vi "Dashboard Main.vi"() -> ()   [LabVIEW 2015]
uses:
  <vilib>/event_ctls.llb/eventvkey.ctl
  <vilib>/Utility/config.llb/NI_LVConfig.lvlib
  <vilib>/Utility/config.llb/Write Key (I32).vi
  <vilib>/Rock Robotics/WPI/Dashboard/WPI_DashboardLogging Global.vi
  <vilib>/Utility/config.llb/Write Key (String).vi
  <vilib>/Rock Robotics/Network Tables/NT Read Numeric Array.vi
  <vilib>/Utility/miscctls.llb/LVRowAndColumnTypeDef.ctl
  <vilib>/Rock Robotics/Network Tables/NT Write Boolean.vi
  <vilib>/Rock Robotics/Network Tables/NT Read Boolean.vi
panel:
  in  "TCP":refnum<k5>
  in  "Rec Mode":enum32{"Stop", "Record", "Playback"}(radio)
  in  "Vision":u16(ring) items=["Camera Off", "USB Camera SW", "USB Camera HW", "IP Camera"]
  out "Camera IP":string
  out "Image Message":string="Timeout in Camera Communications"
  in  "Dashboard Tab":T1(tab)
  in  "Select Auto":string(combo)
  out "NT Connection":bool
  in  "Camera Settings":T2={"Frame Rate"=30, "Compression"=30, "Size"=1} {"Frame Rate" scale=1.0..30.0; "Size" items=["640x480", "320x240", "160x120"]}
  out "MotorChart R":cluster{"Numeric":dbl, "Numeric":dbl}(graph)
  out "MotorChart L":T3(graph)
  out "MotorSliders R":cluster{"MotorSlide1":dbl, "MotorSlide2":dbl} {"MotorSlide2" scale=-1.0..1.0 scale format="%#_2e"; "MotorSlide1" scale=-1.0..1.0 scale format="%#_2e"}
  out "MotorSliders L":T4 {"MotorSlide4 2" scale=0.0..14.0 scale format="%#_2e"; "MotorSlide2" scale=-1.0..1.0 scale format="%#_2e"; "MotorSlide1" scale=-1.0..1.0 scale format="%#_2e"}
  out "Gyro":dbl(knob) scale=0.0..360.0
  out "JS1 Z":dbl(slide) scale=-1.0..1.0 scale format="%#_2e"
  out "JS1 Graph":cluster{"X":dbl, "Y":dbl}[](graph)
  out "JS1 Buttons":T5
  out "JS2 Z":dbl(slide) scale=-1.0..1.0 scale format="%#_2e"
  out "JS2 Graph":cluster{"X":dbl, "Y":dbl}[](graph)
  out "JS2 Buttons":T5
  out "Mode":T6(ring)=enum."Auto Disabled"
  in  "DB Camera Config":bool
  out "fps":dbl format="%#.1g"
  out "Mbps":dbl format="%#.1g"
  out "Mbps LED":bool
  in  "DB/String 9":string
  in  "DB/String 8":string
  in  "DB/String 7":string
  in  "DB/String 6":string
  in  "DB/String 5":string
  in  "DB/String 4":string
  in  "DB/String 3":string
  in  "DB/String 2":string
  in  "DB/String 1":string
  in  "DB/String 0":string
  in  "DB/Slider 0":dbl(slide) scale=0.0..5.0
  in  "DB/Slider 1":dbl(slide) scale=0.0..5.0
  in  "DB/Slider 2":dbl(slide) scale=0.0..5.0
  in  "DB/Slider 3":dbl(slide) scale=0.0..5.0
  out "DB/LED 3":bool
  out "DB/LED 2":bool
  out "DB/LED 1":bool
  out "DB/LED 0":bool
  in  "DB/Button 3":bool
  in  "DB/Button 2":bool
  in  "DB/Button 1":bool
  in  "DB/Button 0":bool caption="New Name"
  out "Meow2":bool
  in  "Meow":bool
  in  "Test Slider":dbl(slide) scale=0.0..100.0 scale format="%#_3g"
  in  "On/Off":bool caption="Solenoid"
  in  "Test Name":u16(ring) items=["Select the test to run..."]
  in  "Test Tree":string(tree)
  in  "Motor":cluster{"Value":dbl, "Enable":bool} {"Value" scale=-1.0..1.0 scale format="%#_3g"}
  out "Progress":T7 {"Test Progress" scale=0.0..100.0}
  in  "Rev/Fwd":cluster{"Forward":bool, "Reverse":bool}
  in  "Test Ring":u16(ring) items=["Monochrome", "Color"]
  out "Cmd Status":string
  in  "Execute Command":bool
  in  "Command Params":string[][](table)
  in  "Command Selection":i32(listbox)
  in  "CheckList":i32(listbox)
  out "Tree":string(tree)
  out "Camera Image":T8(plugin-control)
  out "Background":bool
  # "Left"
  # "Front"
  # "Right"
  # "Battery"
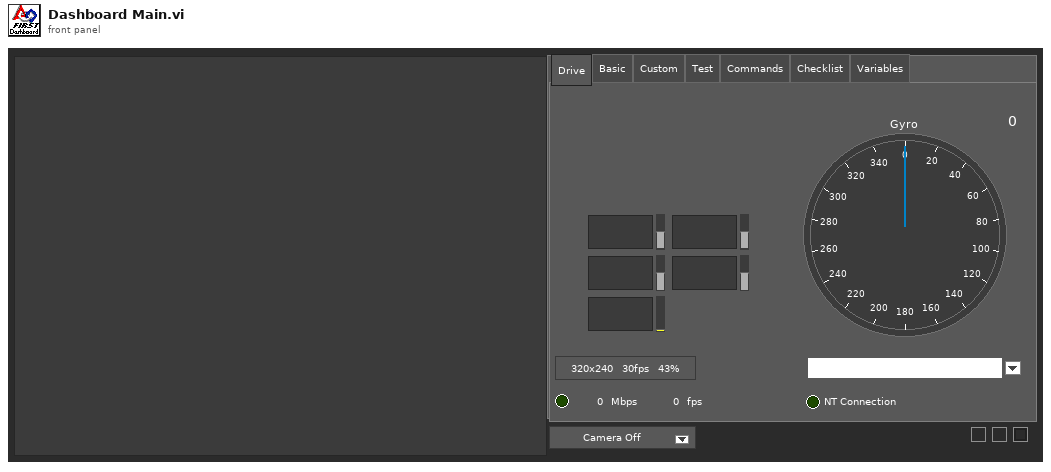
[diagram p1: front panel]
types:
  T1 = enum32{"Drive", "Basic", "Custom", "Test", "Commands", "Checklist", "Variables"}
  T2 = cluster{"Frame Rate":i32, "Compression":i32, "Size":u16}
  T3 = cluster{"Numeric":dbl, "Numeric":dbl, "Battery V":dbl}
  T4 = cluster{"MotorSlide1":dbl, "MotorSlide2":dbl, "MotorSlide4 2":dbl}
  T5 = cluster{bool, bool, bool, bool, bool, bool, bool, bool, bool, bool, bool, bool}
  T6 = enum8{"Tele-Op Disabled", "Tele-Op Enabled", "Auto Disabled", "Auto Enabled", "Test Disabled", "Test Enabled", "Disconnected", "No Code", "E-Stop"}
  T7 = cluster{"Test Progress":u8, "Test Progress Text":string}
  T8 = typedef "IMAQ Image.ctl" = refnum<image>
  T9 = cluster{"IDs":cluster{"RPC field ID":u16, "Unique ID":u16}, "String":string}
  T10 = enum32{"Drive", "Basic", "Custom", "Test", "Checklist", "Variables"}
  T11 = typedef "Image Type" = u32
  T12 = cluster{"Camera Image":refnum<vi>, "Dashboard Tab":refnum<vi>, "Background":refnum<vi>, "Vision":refnum<vi>, "Rec Mode":refnum<vi>, "Test Slider":refnum<vi>, "On/Off ":refnum<vi>, "Test Ring":refnum<vi>, "Rev/Fwd":refnum<vi>, "Test Name":refnum<vi>, "Motor":refnum<vi>, "Progress":refnum<vi>, "CheckList":refnum<vi>, "Tree":refnum<vi>, "Test Tree":refnum<vi>, "Command Params":refnum<vi>, "Command Selection":refnum<vi>, "Execute Command":refnum<vi>, "Cmd Status":refnum<vi>}
  T13 = cluster{"Error Strings":string, "Disable Counts":cluster{u16, u16}, "Rail Faults":cluster{u16, u16, u16}, "Robot IP":string, "DB Mode":u8, "Event Info":cluster{"Name":string, "Type":u8, "Number":u16, "Replay":u8}, "Camera Addr":string}
  T14 = cluster{"Storage":cluster{"Disk Free":u64, "RAM Block":u32, "RAM free":u32}, "CPU Utilization":cluster{"CPU % ISR":sgl, "CPU % Time Crit":sgl, "CPU % Timed Str":sgl, "CPU % High":sgl, "CPU % Above":sgl, "CPU % Normal":sgl, "CPU % Low":sgl}, "CAN":cluster{"% Bus Utilization":sgl, "Bus Off Cnt":u32, "TX_FIFO Full Cnt":u32, "Receive Error Cnt":u8, "Transmit Error Cnt":u8}, "HID":cluster{"HID Outputs":u32, "Rumble Low":u16, "Rumble High":u16}[]}
  T15 = cluster{"Status bits":cluster{"Test Mode":bool, "Autonomous":bool, "Enabled":bool, "Code Start":bool, "Brownout":bool, "Reserved 2":bool, "Reserved 3":bool, "E-Stop":bool}, "Code Trace":cluster{"Disabled":bool, "TeleOp":bool, "Auto":bool, "Test":bool}, "Controller Type":enum16{"unknown", "cRIO", "roboRio"}, "Code?":enum16{"unknown", "noCode", "code"}, "Battery V":dbl}
  T16 = cluster{"Control Bits":cluster{"TestMode":bool, "Autonomous":bool, "Enabled":bool, "FMS Present":bool, bool, bool, bool, "E-Stop":bool}, "Team Station ":u8, "Countdown":sgl, "Joystick Values":cluster{"Axes":dbl[], "Buttons":bool[], "POVs":i16[]}[]}
  T17 = cluster{"Axes":dbl[], "Buttons":bool[], "POVs":i16[]}[]
  T18 = cluster{"Axes":dbl[], "Buttons":bool[], "POVs":i16[]}
  T19 = cluster{"Buttons[0]":bool, "Buttons[1]":bool, "Buttons[2]":bool, "Buttons[3]":bool, "Buttons[4]":bool, "Buttons[5]":bool, "Buttons[6]":bool, "Buttons[7]":bool, "Buttons[8]":bool, "Buttons[9]":bool, "Buttons[10]":bool, "Buttons[11]":bool}
  T20 = typedef "NI_LVConfig.lvlib/Config Data RefNum.ctl" = refnum<k1>
  T21 = cluster{"Operation":enum16{"Update", "Clear"}, "Color Box":u32}[]
  T22 = typedef "eventvkey.ctl" = enum16{"ASCII", "Enter", "Return", "Shift", "Ctrl", "Alt", "Cmd", "Opt", "Caps", "NumLock", "Clear", "Break", "Up", "Down", "Left", "Right", "Insert", "Delete", "Home", "End", "PageUp", "PageDown", "Escape", "Help", "Pause", "ScrollLock", "F1", "F2", "F3", "F4", "F5", "F6", "F7", "F8", "F9", "F10", "F11", "F12", "F13", "F14", "F15", "F16", "F17", "F18", "F19", "F20", "F21", "F22", "F23", "F24", "Play", "VolumeUp", "VolumeDown", "Mute", "Two Byte Char"}
  T23 = cluster{"Image Size":bool, "Image Type":bool, "Pixel Value":bool, "ROI Information":bool, "Zoom Factor":bool}
  T24 = enum8{"Enabled", "Disabled", "Disabled and Grayed Out"}
  T25 = cluster{"Operation":enum16{"Update", "Clear"}, "Color Box":u32}
  T26 = typedef "LVRowAndColumnTypeDef.ctl" = cluster{"Row":i32, "Column":i32}
  T27 = cluster{"Shift":bool, "Ctrl":bool, "Alt":bool, "Cmd":bool, "Opt":bool}
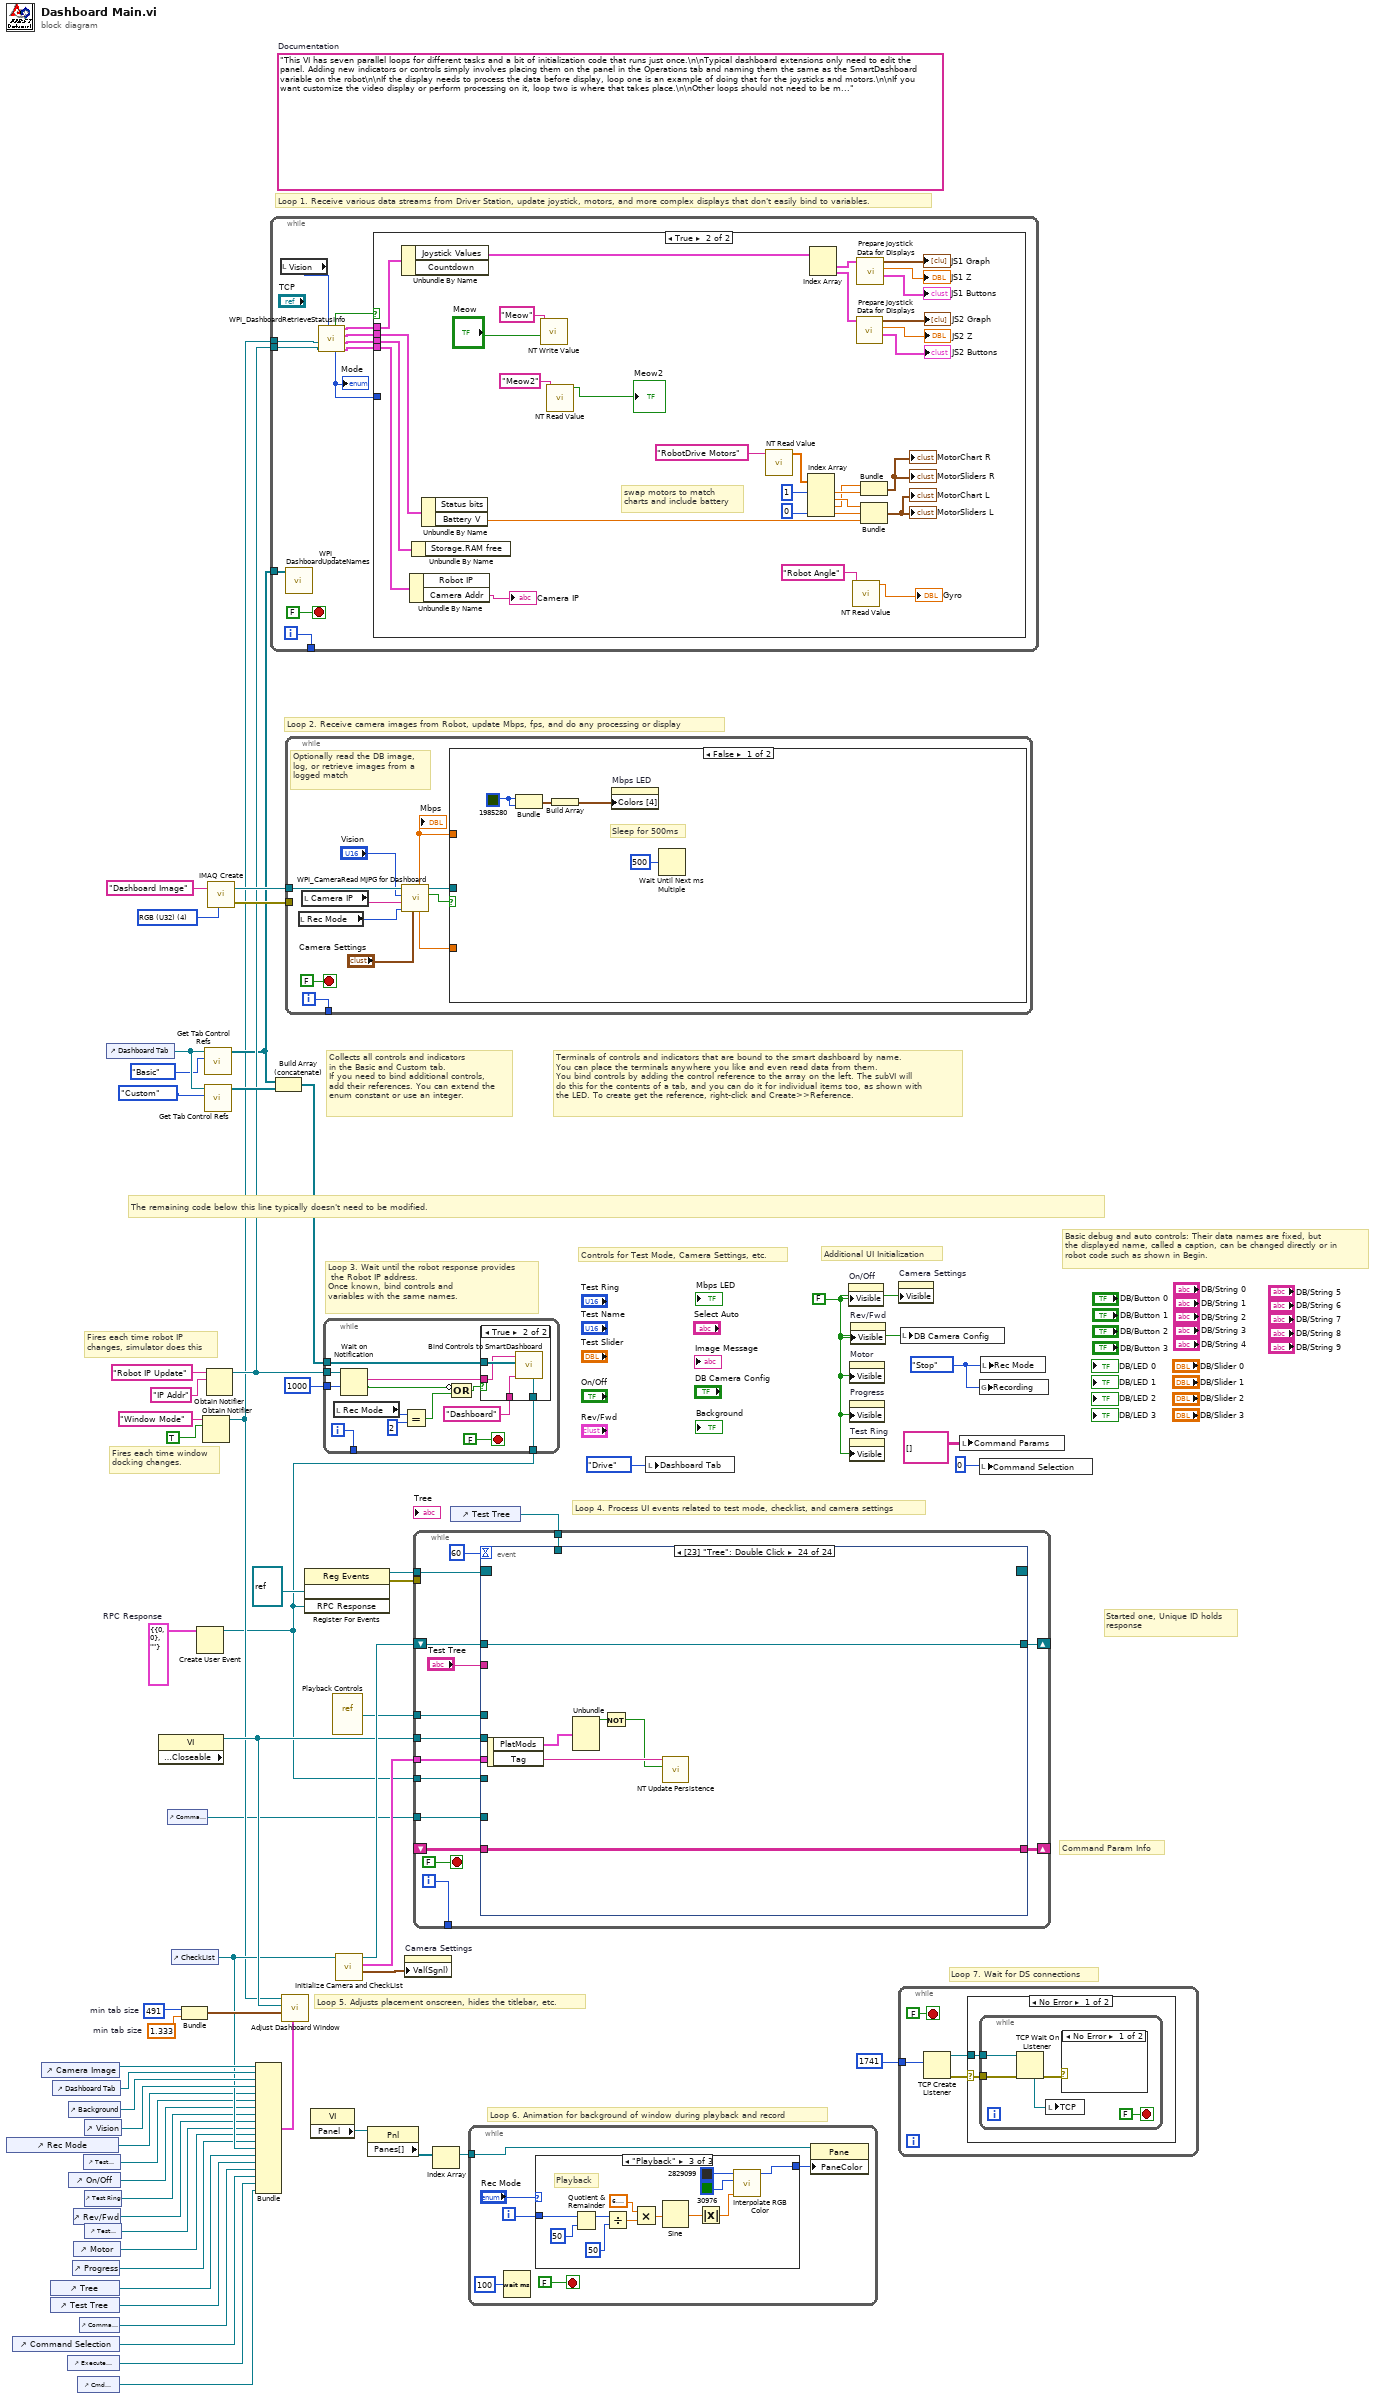
[diagram p0: block diagram]
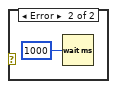
[diagram p2: hidden frame]
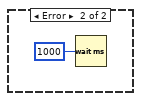
[diagram p3: hidden frame]
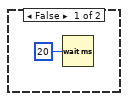
[diagram p4: hidden frame]
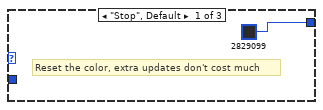
[diagram p5: hidden frame]
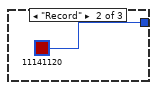
[diagram p6: hidden frame]
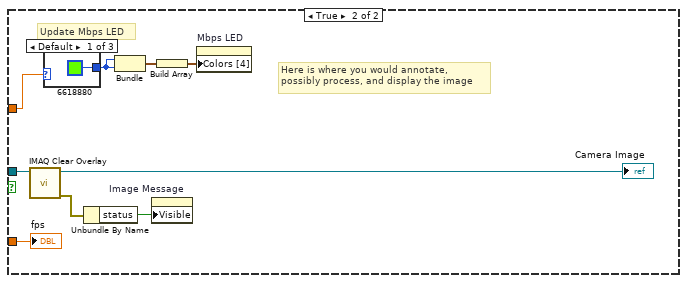
[diagram p8: hidden frame]
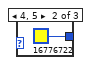
[diagram p9: hidden frame]
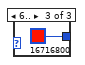
[diagram p10: hidden frame]
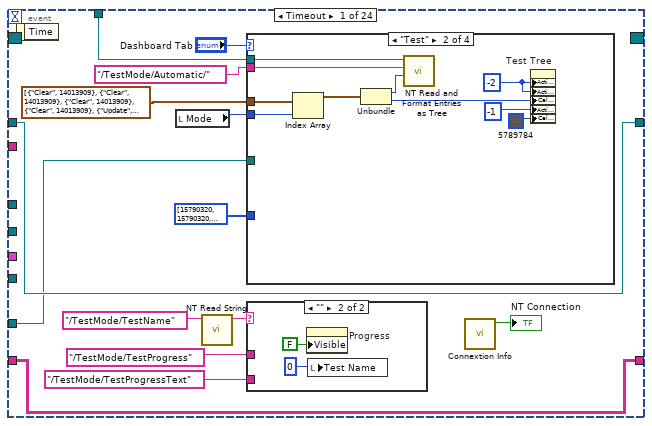
[diagram p11: hidden frame]
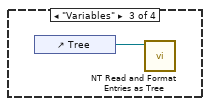
[diagram p13: hidden frame]
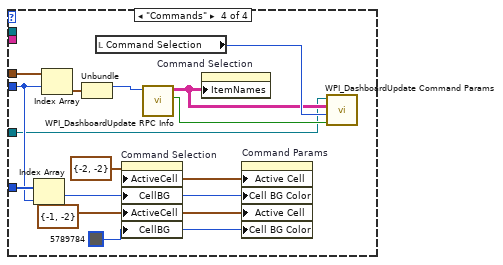
[diagram p14: hidden frame]
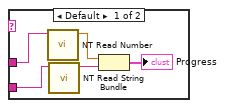
[diagram p15: hidden frame]
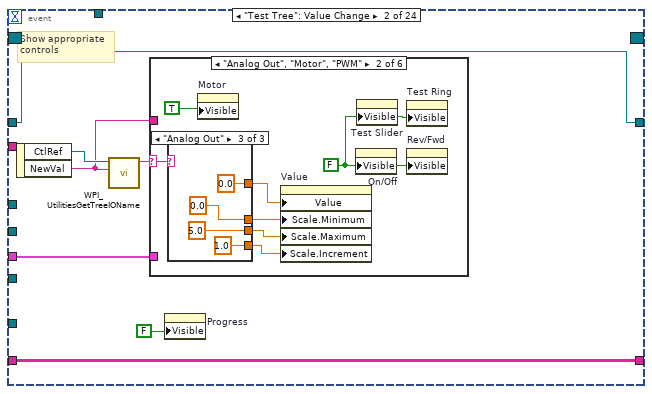
[diagram p16: hidden frame]
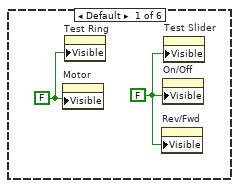
[diagram p17: hidden frame]
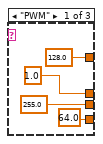
[diagram p18: hidden frame]
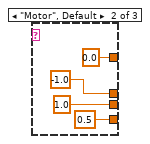
[diagram p19: hidden frame]
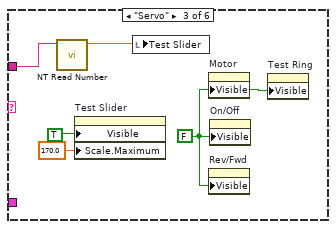
[diagram p20: hidden frame]
diagram:
  w7 = T9 {"IDs"={"RPC field ID"=0, "Unique ID"=0}, "String"=""}  # RPC Response
  w33 = 491  # min tab size
  w32 = 1.333  # min tab size
  w41 = enum32{"Stop", "Record", "Playback"}."Stop" ("Rec Mode")
  w15 = FALSE ("Visible")
  (unwired) "This VI has seven parallel loops for different tasks and a bit of initialization code that runs just once.\n\nTypical dashboard extensions only need to edit the panel. Adding new indicators or controls simply involves placing them on the panel in the Operations tab and naming them the same as the SmartDashboard variable on the robot\n\nIf the display needs to process the data before display, loop one is an example of doing that for the joysticks and motors.\n\nIf you want customize the video display or perform processing on it, loop two is where that takes place.\n\nOther loops should not need to be modified. They are pretty standard, and document the task they perform."  # Documentation
  w61 = T11 4 items=["Grayscale (U8)", "Grayscale (I16)", "Grayscale (SGL)", "Complex (CSG)", "RGB (U32)", "HSL (U32)", "RGB (U64)"] ("Image Type")
  # "Command Param Info"
  # "Started one, Unique ID holds\nresponse"
  # "Loop 7. Wait for DS connections"
  # "Basic debug and auto controls: Their data names are fixed, but\nthe displayed name, called a caption, can be changed directly or in\nrobot code such as shown in Begin."
  # "Controls for Test Mode, Camera Settings, etc."
  # "Additional UI Initialization"
  # "Loop 6. Animation for background of window during playback and record"
  # "Fires each time robot IP\nchanges, simulator does this"
  # "Fires each time window\ndocking changes."
  # "Collects all controls and indicators\nin the Basic and Custom tab.\nIf you need to bind additional controls,\nadd their references. You can extend the\nenum constant or use an integer."
  # "The remaining code below this line typically doesn't need to be modified."
  # "Loop 4. Process UI events related to test mode, checklist, and camera settings"
  # "Terminals of controls and indicators that are bound to the smart dashboard by name.\nYou can place the terminals anywhere you like and even read data from them.\nYou bind controls by adding the control reference to the array on the left. The subVI will\ndo this for the contents of a tab, and you can do it for individual items too, as shown with\nthe LED. To create get the reference, right-click and Create>>Reference."
  # "Loop 3. Wait until the robot response provides\n the Robot IP address.\nOnce known, bind controls and\nvariables with the same names."
  # "Loop 5. Adjusts placement onscreen, hides the titlebar, etc."
  # "Loop 1. Receive various data streams from Driver Station, update joystick, motors, and more complex displays that don't easily bind to variables."
  # "Loop 2. Receive camera images from Robot, update Mbps, fps, and do any processing or display"
  n1 = control-ref of="Rec Mode"() -> (w21:refnum<vi>)
  n2 = control-ref of="Command Selection"() -> (w6:refnum<vi>)
  n3 = control-ref of="Camera Image"() -> (w36:refnum<vi>)
  n4 = control-ref of="Tree"() -> (w25:refnum<vi>)
  n5 = control-ref of="Test Tree"() -> (w24:refnum<vi>)
  n6 = control-ref of="Dashboard Tab"() -> (w35:refnum<vi>)
  n7 = control-ref of="Execute Command"() -> (w8:refnum<vi>)
  n8 = control-ref of="Background"() -> (w30:refnum<vi>)
  n9 = control-ref of="On/Off"() -> (w19:refnum<vi>)
  n10 = control-ref of="Progress"() -> (w16:refnum<vi>)
  n11 = control-ref of="Rev/Fwd"() -> (w17:refnum<vi>)
  n12 = control-ref of="Motor"() -> (w22:refnum<vi>)
  n13 = control-ref of="Cmd Status"() -> (w2:refnum<vi>)
  n14 = control-ref of="Command Params"() -> (w9:refnum<vi>)
  n15 = control-ref of="Test Slider"() -> (w20:refnum<vi>)
  n16 = control-ref of="Vision"() -> (w34:refnum<vi>)
  n17 = control-ref of="Test Ring"() -> (w18:refnum<vi>)
  n18 = control-ref of="Test Name"() -> (w23:refnum<vi>)
  n19 = control-ref of="Dashboard Tab"() -> (w39:refnum<vi>)
  n20 = property class="VI" props=["Front Panel.Closeable"]() -> (reference out=w40:refnum<vi>)  [unwired: 2 in, 2 out]
  n21 = control-ref of="Command Params"() -> (w1:refnum<vi>)
  n22 = control-ref of="CheckList"() -> (w26:refnum<vi>)
  n23 = Bundle("min tab size"=w33, "min tab size"=w32) -> (w31:cluster{"min tab size":i32, "min tab size":dbl})  [unwired: 1 in]
  n24 = Create User Event(user event datatype=w7) -> (user event=w3:refnum<user-event>)  [unwired: 1 in, 1 out]
  n25 = Obtain Notifier(name (unnamed)="Window Mode", notification data type=TRUE) -> (notifier out=w12:refnum<notifier>)  [unwired: 2 in, 2 out]
  n26 = call <vilib>:"Get Tab Control Refs.vi"("Page Index"=T10."Basic" ("Dashboard Tab"), "TabControl in"=w39) -> ("ControlsOnPage"=w13:refnum<vi>[])  [unwired: 9 in]
  n27 = call <vilib>:"Get Tab Control Refs.vi"("Page Index"=T10."Custom" ("Dashboard Tab"), "TabControl in"=w39) -> ("ControlsOnPage"=w38:refnum<vi>[])  [unwired: 9 in]
  n28 = Obtain Notifier(name (unnamed)="Robot IP Update", notification data type="IP Addr" ("name (unnamed)")) -> (notifier out=w14:refnum<notifier>)  [unwired: 2 in, 2 out]
  n29 = call "IMAQ Create"("Image Name"="Dashboard Image", "Image Type"=w61) -> ("New Image"=w59:T8, "error out"=w58:errorcluster)  [unwired: 2 in, 1 out]
  n30 = Bundle("Camera Image"=w36, "Dashboard Tab"=w35, "Background"=w30, "Vision"=w34, "Rec Mode"=w21, "Test Slider"=w20, "On/Off"=w19, "Test Ring"=w18, "Rev/Fwd"=w17, "Test Name"=w23, "Motor"=w22, "Progress"=w16, "CheckList"=w26, "Tree"=w25, "Test Tree"=w24, "Command Params"=w9, "Command Selection"=w6, "Execute Command"=w8, "Cmd Status"=w2) -> (w27:T12)  [unwired: 1 in]
  n31 = while {
    tunnel: [w72] -> _
    tunnel: w14 -> [w63]
    tunnel: w13 -> [w71]
    tunnel: w12 -> [w62]
    i -> [w72]
    stop <- FALSE stop-if-true
    n32 = local read "Vision"() -> (w70:u16)
    n33 = call <vilib>:"WPI_DashboardUpdateNames.vi"("Controls on Tab"=w71) -> ()  [unwired: 11 in]
    n34 = call <vilib>:"WPI_DashboardRetrieveStatusInfo.vi"("Vision"=w70, "Binding Refnum"=w63, "Window Mode Notifier"=w62) -> ("Power and Errors"=w65:T13, "Robot Metrics"=w66:T14, "Status Info"=w67:T15, "Control Info"=w68:T16, "Robot Mode"=w64:T6, "Process?"=w69:bool)  [unwired: 3 in]
    "Mode" <- w64
    n35 = case shown="True" w69 {
      tunnel: w67 -> [_ w105]
      tunnel: w66 -> [_ w104]
      tunnel: w68 -> [_ w103]
      tunnel: w65 -> [_ w102]
      tunnel: w64 -> [_ _]
      frame False {
        n36 = Wait (ms)(milliseconds to wait=u32 20) -> ()  [unwired: 1 out]
      }
      frame True {
        # "swap motors to match\ncharts and include battery"
        n37 = Unbundle By Name(w103) -> ("Joystick Values"=w92:T17)  [unwired: 1 out]
        n38 = Unbundle By Name(w102) -> ("Camera Addr"=→"Camera IP":string)  [unwired: 1 out]
        n39 = Unbundle By Name(w104) -> ()  [unwired: 1 out]
        n40 = Unbundle By Name(w105) -> ("Battery V"=w93:dbl)  [unwired: 1 out]
        n41 = call-poly <vilib>:"NT Write Value.vi"("Boolean"="Meow", "Name"="Meow") -> ()  [unwired: 9 in, 1 out]
        n42 = call-poly <vilib>:"NT Read Value.vi"("Name"="Meow2") -> ("Boolean"=→"Meow2":bool)  [unwired: 9 in, 1 out]
        n43 = call-poly <vilib>:"NT Read Value.vi"("Name"="RobotDrive Motors") -> ("Numeric Array"=w81:dbl[])  [unwired: 9 in, 1 out]
        n44 = Index Array(array=w81, index #1=1, index #4=0) -> (element #1=w97:dbl, element #2=w98:dbl, element #3=w96:dbl, element #4=w101:dbl)  [unwired: 2 in]
        n45 = Index Array(array=w92) -> (element #1=w91:T18, element #2=w86:T18)  [unwired: 2 in]
        n46 = call-poly <vilib>:"NT Read Value.vi"("Name"="Robot Angle") -> ("Numeric"=→"Gyro":dbl)  [unwired: 9 in, 1 out]
        n47 = call "Prepare Joystick Data for Displays.vi"("Joystick Values"=w86) -> ("Buttons"=→"JS2 Buttons":T19, "Z Axis"=→"JS2 Z":dbl, "Cartesian Data"=→"JS2 Graph":cluster{"X axis":dbl, "X axis":dbl}[])  [unwired: 8 in]
        n48 = call "Prepare Joystick Data for Displays.vi"("Joystick Values"=w91) -> ("Buttons"=→"JS1 Buttons":T19, "Z Axis"=→"JS1 Z":dbl, "Cartesian Data"=→"JS1 Graph":cluster{"X axis":dbl, "X axis":dbl}[])  [unwired: 8 in]
        n49 = Bundle("Numeric"=w96, "Numeric"=w97) -> (→"MotorChart R" →"MotorSliders R":cluster{"Numeric":dbl, "Numeric":dbl})  [unwired: 1 in]
        n50 = Bundle("Numeric"=w98, "Numeric"=w101, "Battery V"=w93) -> (→"MotorChart L" →"MotorSliders L":T3)  [unwired: 1 in]
      }
    }
  }
  n51 = Build Array (concatenate)(w13, w38) -> (w37:refnum<vi>[])
  n52 = call "Adjust Dashboard Window.vi"("Sizing Refnums"=w27, "Size Constraints"=w31, "VI"=w40, "WIn Mode"=w12) -> ()  [unwired: 8 in]
  n53 = while {
    tunnel: w59 -> [w114]
    tunnel: w58 -> [_]
    tunnel: [w115] -> _
    i -> [w115]
    stop <- FALSE stop-if-true
    # "Optionally read the DB image,\nlog, or retrieve images from a\nlogged match"
    n54 = local read "Rec Mode"() -> (w109:enum32{"Stop", "Record", "Playback"})
    n55 = local read "Camera IP"() -> (w107:string)
    n56 = call <vilib>:"WPI_CameraRead MJPG for Dashboard.vi"("Camera Settings"="Camera Settings", "Rec Mode"=w109, "Camera IP"=w107, "Camera Mode"="Vision", "Refnum in"=w114) -> ("Active"=w112:bool, "Refnum out"=w113:T8, "FPS"=w111:dbl, "Bandwidth (Mbps)"=w106:dbl)  [unwired: 3 in]
    "Mbps" <- w106
    n57 = case shown="False" w112 {
      tunnel: w113 -> [_ w124]
      tunnel: w106 -> [_ w123]
      tunnel: w111 -> [_ w121]
      frame False {
        w117 = u32 1985280 ("Color Box")
        # "Sleep for 500ms"
        n58 = Bundle("Color Box"=w117, "Color Box"=w117) -> (w119:cluster{"Color Box":u32, "Color Box":u32})  [unwired: 1 out]
        n59 = Build Array(w119) -> (w118:cluster{"Color Box":u32, "Color Box":u32}[])
        n60 = property on="Mbps LED" class="Bool (strict)"("Colors [4]"=w118) -> ()  [unwired: 2 in, 2 out]
        n61 = Wait Until Next ms Multiple(millisecond multiple=u32 500) -> ()  [unwired: 1 out]
      }
      frame True {
        # "Here is where you would annotate,\npossibly process, and display the image"
        # "Update Mbps LED"
        n62 = call "IMAQ Clear Overlay"("Image"=w124) -> ("error out"=w128:errorcluster, "Image Out"=→"Camera Image":T8)  [unwired: 2 in, 7 out]
        n63 = case shown="Default" w123 {
          tunnel: [u32 6618880 ("Color Box") u32 16776722 ("Color Box") u32 16716800 ("Color Box")] -> w125
          frame Default {
          }
          frame 4, 5 {
          }
          frame 6.. {
          }
        }
        n64 = Unbundle By Name(w128) -> ("status"=w129:bool)
        n65 = Bundle("Color Box"=w125, "Color Box"=w125) -> (w127:cluster{"Color Box":u32, "Color Box":u32})  [unwired: 1 out]
        n66 = property on="Image Message" class="Str"("Visible"=w129) -> ()  [unwired: 2 in, 2 out]
        n67 = Build Array(w127) -> (w126:cluster{"Color Box":u32, "Color Box":u32}[])
        n68 = property on="Mbps LED" class="Bool (strict)"("Colors [4]"=w126) -> ()  [unwired: 2 in, 2 out]
        "fps" <- w121
      }
    }
  }
  n69 = register-events(refnum<vi> refnum, w3) -> (reference out=w45:refnum<event-registration>, error out=w44:errorcluster)  [unwired: 2 in]
  n70 = property class="VI"() -> ("Panel"=w48:refnum<vi>)  [unwired: 2 in, 2 out]
  n71 = while {
    tunnel: w37 -> [w145]
    tunnel: w14 -> [w143]
    tunnel: [w141] -> _
    tunnel: u32 1000 ("milliseconds to wait") -> [w140]
    tunnel: w3 -> [w133]
    i -> [w141]
    stop <- FALSE stop-if-true
    n72 = local read "Rec Mode"() -> (w136:enum32{"Stop", "Record", "Playback"})
    n73 = Wait on Notification(notifier=w143, timeout in ms (-1)=w140) -> (notification=w142:string, timed out?=w138:bool)  [unwired: 2 in, 2 out]
    n74 = Equal?(x=w136, y=u16 2 ("Rec Mode")) -> (x = y?=w137:bool)
    n75 = Compound Arithmetic op=OR(invert w138, w137) -> (w139:bool)
    n76 = case shown="True" w139 {
      tunnel: w145 -> [_ w149]
      tunnel: w142 -> [_ w148]
      tunnel: "Dashboard" -> [_ w147]
      tunnel: w133 -> [_ w146]
      frame False {
      }
      frame True {
        n77 = call <vilib>:"Bind Controls to SmartDashboard.vi"("RPC ref"=w146, "Client Name"=w147, "Bound Control Refs"=w149, "Server IP Address"=w148) -> ()  [unwired: 8 in]
      }
    }
  }
  n78 = vi-ref "Playback Controls.vi"() -> (w46:refnum<vi>)
  n79 = call "Initialize Camera and CheckList.vi"("ListBox in"=w26) -> ("Cluster"=w52:cluster{"value":i32, "value":i32, "index":i32}, "Array"=w53:cluster{string[]}[], "File Refnum"=w51:T20)  [unwired: 8 in]
  n80 = property class="Pnl"(reference=w48) -> ("Panes[]"=w49:refnum<vi>[])  [unwired: 1 in, 2 out]
  n81 = property on="Camera Settings" class="Clust (strict)"("Val(Sgnl)"=w52) -> ()  [unwired: 2 in, 2 out]
  n82 = Index Array(array=w49) -> (element=w47:refnum<vi>)  [unwired: 1 in]
  n83 = control-ref of="Test Tree"() -> (w50:refnum<vi>)
  n84 = while {
    tunnel: w53 -> [w161]
    shift-right: [w160] -> _
    shift-left: w51 -> [w159]
    tunnel: [w158] -> _
    tunnel: w50 -> [w157]
    tunnel: w46 -> [w156]
    tunnel: w45 -> [w155]
    tunnel: w44 -> [_]
    tunnel: w40 -> [w154]
    tunnel: w3 -> [w153]
    tunnel: w1 -> [w152]
    shift-right: [w151] -> _
    shift-left: _ -> [w150]
    i -> [w158]
    stop <- FALSE stop-if-true
    n85 = event shown="[23] \"Tree\": Double Click" {
      selector: w155 -> [_ _ _ _ _ _ _ _ _ _ _ _ _ _ _ _ _ _ _ _ _ _ _ _]
      dyn-events: [_ _ _ _ _ _ _ _ _ _ _ _ _ _ _ _ _ _ w470 _ _ _ _ _] -> _
      timeout: u32 60 ("milliseconds to wait") -> [_ _ _ _ _ _ _ _ _ _ _ _ _ _ _ _ _ _ _ _ _ _ _ _]
      tunnel: w157 -> [w174 _ _ _ _ _ _ _ _ _ _ _ _ _ _ _ _ _ _ _ _ _ _ _]
      tunnel: "Test Tree" -> [_ _ _ _ _ _ _ _ _ _ _ _ _ w433 w442 w445 w450 w459 _ _ _ _ _ _]
      tunnel: w161 -> [_ w212 _ _ _ _ _ _ _ _ _ w395 w426 _ _ _ _ _ _ _ _ _ _ _]
      tunnel: [w171 w211 w315 w321 w331 w335 w341 w353 w361 w367 w380 w394 w419 w432 w440 w444 w449 w458 w472 w488 w490 w498 w509 w514] -> w160
      tunnel: w159 -> [w171 w211 w315 w321 w331 w335 w341 w353 w361 w367 w380 w393 w419 w432 w440 w444 w449 w458 w472 w488 w490 w498 w509 w514]
      tunnel: w156 -> [_ _ _ _ _ _ _ _ _ _ _ _ _ _ _ _ _ _ w473 _ w493 _ _ _]
      tunnel: w154 -> [_ _ _ _ _ _ _ _ _ _ _ _ _ _ _ _ _ _ w468 _ _ _ _ _]
      tunnel: w153 -> [_ _ _ _ _ _ _ _ _ _ _ _ _ _ _ _ _ _ w464 _ _ _ _ _]
      tunnel: w152 -> [w166 _ _ _ _ _ w339 _ _ _ _ _ _ _ _ _ _ _ _ _ _ _ _ _]
      tunnel: [w165 w210 w314 w320 w330 w336 w337 w347 w358 w366 w379 w392 w418 w431 w439 w443 w448 w457 w463 w486 w489 w494 w502 w515] -> w151
      tunnel: w150 -> [w165 w210 w314 w320 w330 w336 w337 _ _ w366 w379 w392 w418 w431 w439 w443 w448 w457 w463 w486 w489 w494 w502 w515]
      event Timeout {
        n86 = event-data() -> ()  [unwired: 1 in, 1 out]
        n87 = local read "Mode"() -> (w168:T6)
        n88 = call <vilib>:"NT Read String.vi"("Name"="/TestMode/TestName") -> ("String"=w177:string)  [unwired: 9 in, 1 out]
        n89 = case shown="\"Test\"" "Dashboard Tab" {
          tunnel: w174 -> [_ w188 _ _]
          tunnel: "/TestMode/Automatic/" ("Name Pattern") -> [_ w187 _ _]
          tunnel: T21 [{"Operation"=enum."Clear", "Color Box"=14013909}, {"Operation"=enum."Clear", "Color Box"=14013909}, {"Operation"=enum."Clear", "Color Box"=14013909}, {"Operation"=enum."Clear", "Color Box"=14013909}, {"Operation"=enum."Update", "Color Box"=14013909}, {"Operation"=enum."Update", "Color Box"=16777215}, {"Operation"=enum."Clear", "Color Box"=14013909}, {"Operation"=enum."Clear", "Color Box"=14013909}, {"Operation"=enum."Clear", "Color Box"=14013909}] -> [_ w180 _ w197]
          tunnel: w168 -> [_ w179 _ w196]
          tunnel: u32[] [15790320, 15790320, 15790320, 15790320, 16777215, 16777215, 15790320, 15790320, 15790320] -> [_ _ _ w202]
          tunnel: w166 -> [_ _ _ w190]
          frame "Custom", Default {
          }
          frame "Test" {
            w186 = -2 ("Active Item:Row Number")
            n90 = Index Array(array=w180, index=w179) -> (element=w181:T25)
            n91 = Unbundle(w181) -> ("Operation"=w182:enum16{"Update", "Clear"}, "Color Box"=w183:u32)
            n92 = call <vilib>:"NT Read and Format Entries as Tree.vi"("Operation"=w182, "Name Pattern"=w187, "Tree Refnum"=w188) -> ()  [unwired: 7 in, 2 out]
            n93 = property on="Test Tree" class="Tree (strict)"("Active Item Row Number"=w186, "ActiveColNum"=w186, "CellBG"=w183, "Active Item Row Number"=-1 ("Active Item:Row Number"), "CellBG"=u32 5789784 ("Color Box")) -> ()  [unwired: 2 in, 2 out]
          }
          frame "Variables" {
            n94 = control-ref of="Tree"() -> (w189:refnum<vi>)
            n95 = call <vilib>:"NT Read and Format Entries as Tree.vi"("Tree Refnum"=w189) -> ()  [unwired: 9 in, 2 out]
          }
          frame "Commands" {
            w198 = u32 5789784 ("Color Box")
            w199 = T26 {"Row"=-1, "Column"=-2} ("Active Cell:Active Cell")
            w201 = T26 {"Row"=-2, "Column"=-2} ("Active Cell:Active Cell")
            n96 = Index Array(array=w202, index=w196) -> (element=w200:u32)
            n97 = Index Array(array=w197, index=w196) -> (element=w195:T25)
            n98 = Unbundle(w195) -> ("Operation"=w194:enum16{"Update", "Clear"})  [unwired: 1 out]
            n99 = local read "Command Selection"() -> (w193:i32)
            n100 = property on="Command Selection" class="MCListbox (strict)"("ActiveCell"=w201, "CellBG"=w200, "ActiveCell"=w199, "CellBG"=w198) -> ()  [unwired: 2 in, 2 out]
            n101 = call <vilib>:"WPI_DashboardUpdate RPC Info.vi"("Operation"=w194) -> ("update"=w192:bool, "commands"=w191:string[][])  [unwired: 9 in]
            n102 = property on="Command Selection" class="MCListbox (strict)"("ItemNames"=w191) -> ()  [unwired: 2 in, 2 out]
            n103 = property on="Command Params" class="Tbl (strict)"("Active Cell"=w201, "Cell BG Color"=w200, "Active Cell"=w199, "Cell BG Color"=w198) -> ()  [unwired: 2 in, 2 out]
            n104 = call <vilib>:"WPI_DashboardUpdate Command Params.vi"("Update"=w192, "NewVal"=w193, "Commands"=w191, "Param Tbl"=w190) -> ()  [unwired: 7 in, 1 out]
          }
        }
        n105 = case shown="\"\"" w177 {
          tunnel: "/TestMode/TestProgress" ("Name") -> [w204 _]
          tunnel: "/TestMode/TestProgressText" ("Name") -> [w203 _]
          frame Default {
            n106 = call <vilib>:"NT Read Number.vi"("Name"=w204) -> ("Numeric"=w205:dbl)  [unwired: 9 in, 1 out]
            n107 = call <vilib>:"NT Read String.vi"("Name"=w203) -> ("String"=w206:string)  [unwired: 9 in, 1 out]
            n108 = Bundle("Numeric"=w205, "String"=w206) -> (→"Progress":cluster{"Numeric":dbl, "String":string})  [unwired: 1 in]
          }
          frame "" {
            n109 = property on="Progress" class="Clust (strict)"("Visible"=FALSE) -> ()  [unwired: 2 in, 2 out]
            n110 = local write "Test Name"(u16 0) -> ()
          }
        }
        n111 = call <vilib>:"Connextion Info.vi"() -> ("Connected"=→"NT Connection":bool)  [unwired: 10 in, 1 out]
      }
      event "Test Tree": Value Change {
        # "Show appropriate\ncontrols"
        n112 = event-data() -> ("CtlRef"=w215:refnum<vi>, "NewVal"=w213:string)  [unwired: 1 in]
        n113 = call <vilib>:"WPI_UtilitiesGetTreeIOName.vi"("NewVal"=w213, "TreeControl in"=w215) -> ("I/O Name"=w216:string)  [unwired: 9 in]
        n114 = case shown="\"Analog Out\", \"Motor\", \"PWM\"" w216 {
          selector: w216 -> [_ w223 _ w245 w254 _]
          tunnel: w213 -> [_ _ w242 w244 _ w261]
          tunnel: w212 -> [_ _ _ _ _ w260]
          frame Default {
            w218 = FALSE ("Visible")
            w217 = FALSE ("Visible")
            n115 = property on="Motor" class="Clust (strict)"("Visible"=w217) -> ()  [unwired: 2 in, 2 out]
            n116 = property on="Test Ring" class="Ring (strict)"("Visible"=w217) -> ()  [unwired: 2 in, 2 out]
            n117 = property on="Rev/Fwd" class="Clust (strict)"("Visible"=w218) -> ()  [unwired: 2 in, 2 out]
            n118 = property on="On/Off" class="Bool (strict)"("Visible"=w218) -> ()  [unwired: 2 in, 2 out]
            n119 = property on="Test Slider" class="Slide (strict)"("Visible"=w218) -> ()  [unwired: 2 in, 2 out]
          }
          frame "Analog Out", "Motor", "PWM" {
            w224 = FALSE ("Visible")
            n120 = case shown="\"Analog Out\"" w223 {
              tunnel: [1.0 ("Value") -1.0 ("Value") 0.0 ("Value")] -> w222
              tunnel: [255.0 ("Value") 1.0 ("Value") 5.0 ("Value")] -> w221
              tunnel: [128.0 ("Value") 0.0 ("Value") 0.0 ("Value")] -> w220
              tunnel: [64.0 ("Value") 0.5 ("Value") 1.0 ("Value")] -> w219
              frame "PWM" {
              }
              frame "Motor", Default {
              }
              frame "Analog Out" {
              }
            }
            n121 = property on="Motor" class="Clust (strict)"("Visible"=TRUE) -> ()  [unwired: 2 in, 2 out]
            n122 = property on="Value" class="Slide (strict)"("Value"=w220, "Scale.Minimum"=w222, "Scale.Maximum"=w221, "Scale.Increment"=w219) -> ()  [unwired: 2 in, 2 out]
            n123 = property on="On/Off" class="Bool (strict)"("Visible"=w224) -> ()  [unwired: 2 in, 2 out]
            n124 = property on="Test Slider" class="Slide (strict)"("Visible"=w224) -> ()  [unwired: 2 in, 2 out]
            n125 = property on="Test Ring" class="Ring (strict)"("Visible"=w224) -> ()  [unwired: 2 in, 2 out]
            n126 = property on="Rev/Fwd" class="Clust (strict)"("Visible"=w224) -> ()  [unwired: 2 in, 2 out]
          }
          frame "Servo" {
            w240 = FALSE ("Visible")
            n127 = call <vilib>:"NT Read Number.vi"("Name"=w242) -> ("Numeric"=w241:dbl)  [unwired: 9 in, 1 out]
            n128 = property on="Test Slider" class="Slide (strict)"("Visible"=TRUE, "Scale.Maximum"=170.0 ("Scale.Range:Maximum")) -> ()  [unwired: 2 in, 2 out]
            n129 = local write "Test Slider"(w241) -> ()
            n130 = property on="Motor" class="Clust (strict)"("Visible"=w240) -> ()  [unwired: 2 in, 2 out]
            n131 = property on="Rev/Fwd" class="Clust (strict)"("Visible"=w240) -> ()  [unwired: 2 in, 2 out]
            n132 = property on="On/Off" class="Bool (strict)"("Visible"=w240) -> ()  [unwired: 2 in, 2 out]
            n133 = property on="Test Ring" class="Ring (strict)"("Visible"=w240) -> ()  [unwired: 2 in, 2 out]
          }
          frame "Relay", "Solenoid" {
            w243 = FALSE ("Visible")
            n134 = property on="Motor" class="Clust (strict)"("Visible"=w243) -> ()  [unwired: 2 in, 2 out]
            n135 = property on="Test Slider" class="Slide (strict)"("Visible"=w243) -> ()  [unwired: 2 in, 2 out]
            n136 = Search and Replace String(input string=w244, search string="/Value  **", replace string="/Direction") -> (result string=w250:string)  [unwired: 5 in, 3 out]
            n137 = property on="Test Ring" class="Ring (strict)"("Visible"=w243) -> ()  [unwired: 2 in, 2 out]
            n138 = call <vilib>:"NT Read String.vi"("Name"=w250) -> ("String"=w248:string)  [unwired: 9 in, 1 out]
            n139 = Equal?(x="Both directions", y=w248) -> (x = y?=w246:bool)
            n140 = Not(x=w246) -> (.not. x?=w247:bool)
            n141 = property on="Rev/Fwd" class="Clust (strict)"("Visible"=w246) -> ()  [unwired: 2 in, 2 out]
            n142 = property on="On/Off" class="Bool (strict)"("Visible"=w247, "Caption.Text"=w245) -> ()  [unwired: 2 in, 2 out]
          }
          frame "Compressor", "Digital Out" {
            w253 = FALSE ("Visible")
            # "Get direction and finish"
            n143 = property on="Motor" class="Clust (strict)"("Visible"=w253) -> ()  [unwired: 2 in, 2 out]
            n144 = property on="Test Slider" class="Slide (strict)"("Visible"=w253) -> ()  [unwired: 2 in, 2 out]
            n145 = property on="Test Ring" class="Ring (strict)"("Visible"=w253) -> ()  [unwired: 2 in, 2 out]
            n146 = property on="On/Off" class="Bool (strict)"("Visible"=TRUE, "Caption.Text"=w254) -> ()  [unwired: 2 in, 2 out]
            n147 = property on="Rev/Fwd" class="Clust (strict)"("Visible"=FALSE) -> ()  [unwired: 2 in, 2 out]
          }
          frame "Camera" {
            n148 = call <vilib>:"Get Last Path Segment.vi"("String in"=w261) -> ("String out"=w262:string)  [unwired: 10 in]
            n149 = property on="On/Off" class="Bool (strict)"("Visible"=FALSE) -> ()  [unwired: 2 in, 2 out]
            n150 = property on="Motor" class="Clust (strict)"("Visible"=FALSE) -> ()  [unwired: 2 in, 2 out]
            n151 = property on="Rev/Fwd" class="Clust (strict)"("Visible"=FALSE) -> ()  [unwired: 2 in, 2 out]
            n152 = case shown="\"White Balance  **\"" w262 {
              tunnel: w261 -> [w268 w277 w286 w295 w304 _ w310]
              tunnel: w260 -> [w266 w274 w283 w292 w301 _ _]
              frame "Size  **" {
                n153 = Index Array(array=w266) -> (element=w265:cluster{string[]})  [unwired: 1 in]
                n154 = call <vilib>:"NT Read String.vi"("Name"=w268) -> ("String"=w267:string)  [unwired: 9 in, 1 out]
                n155 = Unbundle(w265) -> (w263:string[])
                n156 = Match First String(2:w263, 3:w267) -> (0:w264:i32)  [unwired: 1 out]
                n157 = property on="Test Ring" class="Ring (strict)"("Value"=w264, "Strings []"=w263) -> ()  [unwired: 2 in, 2 out]
                n158 = property on="Test Ring" class="Ring (strict)"("Visible"=TRUE) -> ()  [unwired: 2 in, 2 out]
                n159 = property on="Test Slider" class="Slide (strict)"("Visible"=FALSE) -> ()  [unwired: 2 in, 2 out]
              }
              frame "White Balance  **" {
                n160 = Index Array(array=w274, index=1) -> (element=w275:cluster{string[]})
                n161 = call <vilib>:"NT Read String.vi"("Name"=w277) -> ("String"=w276:string)  [unwired: 9 in, 1 out]
                n162 = Unbundle(w275) -> (w272:string[])
                n163 = Match First String(2:w272, 3:w276) -> (0:w271:i32)  [unwired: 1 out]
                n164 = property on="Test Ring" class="Ring (strict)"("Value"=w271, "Strings []"=w272) -> ()  [unwired: 2 in, 2 out]
                n165 = property on="Test Ring" class="Ring (strict)"("Visible"=TRUE) -> ()  [unwired: 2 in, 2 out]
                n166 = property on="Test Slider" class="Slide (strict)"("Visible"=FALSE) -> ()  [unwired: 2 in, 2 out]
              }
              frame "Exposure  **" {
                n167 = Index Array(array=w283, index=2) -> (element=w284:cluster{string[]})
                n168 = call <vilib>:"NT Read String.vi"("Name"=w286) -> ("String"=w285:string)  [unwired: 9 in, 1 out]
                n169 = Unbundle(w284) -> (w280:string[])
                n170 = Match First String(2:w280, 3:w285) -> (0:w281:i32)  [unwired: 1 out]
                n171 = property on="Test Ring" class="Ring (strict)"("Value"=w281, "Strings []"=w280) -> ()  [unwired: 2 in, 2 out]
                n172 = property on="Test Ring" class="Ring (strict)"("Visible"=TRUE) -> ()  [unwired: 2 in, 2 out]
                n173 = property on="Test Slider" class="Slide (strict)"("Visible"=FALSE) -> ()  [unwired: 2 in, 2 out]
              }
              frame "Exposure Priority  **" {
                n174 = Index Array(array=w292, index=3) -> (element=w293:cluster{string[]})
                n175 = call <vilib>:"NT Read String.vi"("Name"=w295) -> ("String"=w294:string)  [unwired: 9 in, 1 out]
                n176 = Unbundle(w293) -> (w289:string[])
                n177 = Match First String(2:w289, 3:w294) -> (0:w290:i32)  [unwired: 1 out]
                n178 = property on="Test Ring" class="Ring (strict)"("Value"=w290, "Strings []"=w289) -> ()  [unwired: 2 in, 2 out]
                n179 = property on="Test Ring" class="Ring (strict)"("Visible"=TRUE) -> ()  [unwired: 2 in, 2 out]
                n180 = property on="Test Slider" class="Slide (strict)"("Visible"=FALSE) -> ()  [unwired: 2 in, 2 out]
              }
              frame "Color Enable  **" {
                n181 = Index Array(array=w301, index=4) -> (element=w302:cluster{string[]})
                n182 = call <vilib>:"NT Read String.vi"("Name"=w304) -> ("String"=w303:string)  [unwired: 9 in, 1 out]
                n183 = Unbundle(w302) -> (w298:string[])
                n184 = Match First String(2:w298, 3:w303) -> (0:w299:i32)  [unwired: 1 out]
                n185 = property on="Test Ring" class="Ring (strict)"("Value"=w299, "Strings []"=w298) -> ()  [unwired: 2 in, 2 out]
                n186 = property on="Test Ring" class="Ring (strict)"("Visible"=TRUE) -> ()  [unwired: 2 in, 2 out]
                n187 = property on="Test Slider" class="Slide (strict)"("Visible"=FALSE) -> ()  [unwired: 2 in, 2 out]
              }
              frame Default {
                n188 = property on="Test Ring" class="Ring (strict)"("Visible"=FALSE) -> ()  [unwired: 2 in, 2 out]
                n189 = property on="Test Slider" class="Slide (strict)"("Visible"=FALSE) -> ()  [unwired: 2 in, 2 out]
              }
              frame "Brightness  **", "Color Level  **", "Compression  **", "FPS  **", "Sharpness  **" {
                n190 = call <vilib>:"NT Read Number.vi"("Name"=w310) -> ("Numeric"=w309:dbl)  [unwired: 9 in, 1 out]
                n191 = local write "Test Slider"(w309) -> ()
                n192 = property on="Test Slider" class="Slide (strict)"("Visible"=TRUE, "Scale.Maximum"=100.0 ("Scale.Range:Maximum")) -> ()  [unwired: 2 in, 2 out]
                n193 = property on="Test Ring" class="Ring (strict)"("Visible"=FALSE) -> ()  [unwired: 2 in, 2 out]
              }
            }
          }
        }
        n194 = property on="Progress" class="Clust (strict)"("Visible"=FALSE) -> ()  [unwired: 2 in, 2 out]
      }
      event "Test Name": Mouse Enter {
        # "Populate the ring with the list of tests"
        n195 = event-data() -> ()  [unwired: 1 in, 1 out]
        n196 = call <vilib>:"NT Read String Array.vi"("Name"="/TestMode/TestList") -> ("String Array"=w319:string[])  [unwired: 9 in, 1 out]
        n197 = Build Array (concatenate)("Select the test to run...", w319) -> (w318:string[])
        n198 = property on="Test Name" class="Ring (strict)"("Strings []"=w318) -> ()  [unwired: 2 in, 2 out]
      }
      event "Test Name": Value Change {
        w322 = FALSE ("Visible")
        # "Tell the robot the test name to run"
        n199 = event-data() -> ("NewVal"=w326:u16)  [unwired: 1 in]
        n200 = property on="Test Name" class="Ring (strict)"() -> ("Strings []"=w327:string[])  [unwired: 2 in, 2 out]
        n201 = local write "Progress"(T7 {"Test Progress"=0, "Test Progress Text"=""} ("Progress")) -> ()
        n202 = Index Array(array=w327, index=w326) -> (element=w325:string)
        n203 = call <vilib>:"NT Write String.vi"("String"=w325, "Name"="/TestMode/TestName") -> ()  [unwired: 9 in, 1 out]
        n204 = property on="Progress" class="Clust (strict)"("Visible"=TRUE) -> ()  [unwired: 2 in, 2 out]
        n205 = property on="Motor" class="Clust (strict)"("Visible"=w322) -> ()  [unwired: 2 in, 2 out]
        n206 = property on="Test Slider" class="Slide (strict)"("Visible"=w322) -> ()  [unwired: 2 in, 2 out]
        n207 = property on="On/Off" class="Bool (strict)"("Visible"=w322) -> ()  [unwired: 2 in, 2 out]
        n208 = property on="Rev/Fwd" class="Clust (strict)"("Visible"=w322) -> ()  [unwired: 2 in, 2 out]
        n209 = property on="Test Ring" class="Ring (strict)"("Visible"=w322) -> ()  [unwired: 2 in, 2 out]
      }
      event "Select Auto": Mouse Enter {
        # "Populate the combo box with the list of autonomous options"
        n210 = event-data() -> ()  [unwired: 1 in, 1 out]
        n211 = call <vilib>:"NT Read String Array.vi"("Name"="Auto List") -> ("String Array"=w329:string[])  [unwired: 9 in, 1 out]
        n212 = property on="Select Auto" class="CmbBox"("Strings[]"=w329) -> ()  [unwired: 2 in, 2 out]
      }
      event "Select Auto": Value Change {
        # "User modified the Auto Selection. Write to NT variable so robot knows."
        n213 = event-data() -> ("NewVal"=w333:string)  [unwired: 1 in]
        n214 = call <vilib>:"NT Write String.vi"("String"=w333, "Name"="Auto Selector") -> ()  [unwired: 9 in, 1 out]
      }
      event "Command Selection": Value Change {
        # "Get the params and show in table"
        n215 = event-data() -> ("NewVal"=w340:i32)  [unwired: 1 in]
        n216 = property on="Command Selection" class="MCListbox (strict)"() -> ("ItemNames"=w338:string[][])  [unwired: 2 in, 2 out]
        n217 = call <vilib>:"WPI_DashboardUpdate Command Params.vi"("NewVal"=w340, "Commands"=w338, "Param Tbl"=w339) -> ()  [unwired: 8 in, 1 out]
      }
      event "Execute Command": Value Change {
        # "Started one, Unique ID holds\nresponse"
        n218 = event-data() -> ()  [unwired: 1 in, 1 out]
        n219 = property on="Command Selection" class="MCListbox (strict)"() -> ("ItemNames"=w352:string[][])  [unwired: 2 in, 2 out]
        n220 = Index Array(array=w352, index (row)="Command Selection", index (col)=0) -> (element=w350:string)
        n221 = call <vilib>:"Invoke Commands.vi"("Command Params"="Command Params", "Function Name"=w350) -> ("Params"=w346:u8, "Started"=w345:bool)  [unwired: 7 in, 1 out]
        n222 = Array Subset(array="Command Params", length (row)=w346) -> (w347:string[][])  [unwired: 3 in]
        n223 = Select(t="Executing" ("Cmd Status"), s=w345, f="" ("Cmd Status")) -> (s? t:f=→"Cmd Status":string)
      }
      event "Command Selection": Double Click {
        n224 = event-data() -> ("Row"=w362:i32)  [unwired: 1 in]
        n225 = property on="Command Selection" class="MCListbox (strict)"() -> ("ItemNames"=w365:string[][])  [unwired: 2 in, 2 out]
        n226 = local read "Command Params"() -> (w360:string[][])
        n227 = Index Array(array=w365, index (row)=w362, index (col)=0) -> (element=w363:string)
        n228 = call <vilib>:"Invoke Commands.vi"("Command Params"=w360, "Function Name"=w363) -> ("Params"=w359:u8, "Started"=w354:bool)  [unwired: 7 in, 1 out]
        n229 = Array Subset(array=w360, length (row)=w359) -> (w358:string[][])  [unwired: 3 in]
        n230 = Select(t="Executing" ("Cmd Status"), s=w354, f="" ("Cmd Status")) -> (s? t:f=w355:string)
        n231 = local write "Cmd Status"(w355) -> ()
      }
      event "CheckList": Double Click {
        # "Shift clears all"
        # "Update symbols on the listbox"
        n232 = event-data() -> ("PlatMods.Shift"=w368:bool, "Row"=w370:i32)  [unwired: 1 in]
        n233 = case shown="True" w368 {
          tunnel: w370 -> [w374 _]
          tunnel: 1 -> [w373 _]
          frame False {
            n234 = property on="CheckList" class="LstBox (strict)"() -> ("Item Symbols"=w372:i32[])  [unwired: 2 in, 2 out]
            n235 = Replace Array Subset(array=w372, new element=w373, index=w374) -> (w371:i32[])
            n236 = property on="CheckList" class="LstBox (strict)"("Item Symbols"=w371) -> ()  [unwired: 2 in, 2 out]
          }
          frame True {
            w375 = 0 ("Top Row")
            n237 = property on="CheckList" class="LstBox (strict)"() -> ("Number of Rows"=w377:u32)  [unwired: 2 in, 2 out]
            n238 = Initialize Array(0, w377) -> (w376:i32[])
            n239 = property on="CheckList" class="LstBox (strict)"("Top Row"=w375, "Value"=w375, "Item Symbols"=w376) -> ()  [unwired: 2 in, 2 out]
          }
        }
      }
      event "CheckList": Key Down {
        # "Update symbols on the listbox\nLeft and right keys check and uncheck"
        n240 = event-data() -> ("VKey"=w382:T22)  [unwired: 1 in]
        n241 = case shown="\"Left\", \"Right\"" w382 {
          selector: w382 -> [w387 _]
          tunnel: eventvkey."Left" ("VKey") -> [w385 _]
          frame "Left", "Right" {
            n242 = Equal?(x=w385, y=w387) -> (x = y?=w386:bool)
            n243 = Select(t=0, s=w386, f=1) -> (s? t:f=w388:i32)
            n244 = property on="CheckList" class="LstBox (strict)"() -> ("Item Symbols"=w391:i32[])  [unwired: 2 in, 2 out]
            n245 = Replace Array Subset(array=w391, new element=w388, index="CheckList") -> (w390:i32[])
            n246 = property on="CheckList" class="LstBox (strict)"("Item Symbols"=w390) -> ()  [unwired: 2 in, 2 out]
          }
          frame Default {
          }
        }
      }
      event "DB Camera Config": Value Change {
        # "Show or hide the cluster of controls, store in ini file"
        n247 = event-data() -> ("NewVal"=w396:bool)  [unwired: 1 in]
        n248 = case shown="False" w396 {
          tunnel: w395 -> [w405 _]
          tunnel: [w398 w416] -> w394
          tunnel: w393 -> [w397 w416]
          frame False {
            w412 = "Camera"
            w415 = FALSE ("Visible")
            n249 = local read "Camera Settings"() -> (w404:T2)
            n250 = Index Array(array=w405) -> (element=w408:cluster{string[]})  [unwired: 1 in]
            n251 = Unbundle(w404) -> ("Frame Rate"=w403:i32, "Compression"=w402:i32, "Size"=w406:u16)
            n252 = Unbundle(w408) -> (w407:string[])
            n253 = Index Array(array=w407, index=w406) -> (element=w401:string)
            n254 = call-poly <vilib>:"Write Key.vi"("section"=w412, "value"=w401, "key"="Size", "refnum"=w397) -> ("refnum out"=w414:T20)  [unwired: 2 in, 5 out]
            n255 = call-poly <vilib>:"Write Key.vi"("section"=w412, "value"=w403, "key"="FrameRate", "refnum"=w414) -> ("refnum out"=w413:T20)  [unwired: 1 in, 6 out]
            n256 = property on="Camera Settings" class="Clust (strict)"("Visible"=w415) -> ()  [unwired: 2 in, 2 out]
            n257 = local write "DB Camera Config"(w415) -> ()
            n258 = call-poly <vilib>:"Write Key.vi"("section"=w412, "value"=w402, "key"="Compression", "refnum"=w413) -> ("refnum out"=w399:T20)  [unwired: 1 in, 6 out]
            n259 = call <vilib>:"Close Config Data.vi"("refnum"=w399) -> ("file path"=w400:path)  [unwired: 2 in, 8 out]
            n260 = call <vilib>:"Open Config Data.vi"("configuration file path"=w400) -> ("refnum"=w398:T20)  [unwired: 8 in, 2 out]
          }
          frame True {
            n261 = property on="Camera Settings" class="Clust (strict)"("Visible"=TRUE) -> ()  [unwired: 2 in, 2 out]
          }
        }
      }
      event "Camera Settings": Value Change {
        # "Update summary string when any elements of DB camera change"
        n262 = event-data() -> ("NewVal"=w430:T2)  [unwired: 1 in]
        n263 = Index Array(array=w426) -> (element=w425:cluster{string[]})  [unwired: 1 in]
        n264 = Unbundle(w430) -> ("Frame Rate"=w421:i32, "Compression"=w420:i32, "Size"=w423:u16)
        n265 = Unbundle(w425) -> (w424:string[])
        n266 = Index Array(array=w424, index=w423) -> (element=w422:string)
        n267 = Format Into String(format string="%s   %dfps   %d%%", w422, w421, w420) -> (resulting string=w427:string)  [unwired: 2 in, 1 out]
        n268 = Build Array(w427) -> (w428:string[])
        n269 = property on="DB Camera Config" class="Bool (strict)"("Strings [4]"=w428) -> ()  [unwired: 2 in, 2 out]
      }
      event "Motor.Enable": Value Change {
        # "When the test mode otor enable helper is set, update that\ntree row item's value"
        n270 = event-data() -> ("NewVal"=w437:bool)  [unwired: 1 in]
        n271 = Unbundle("Motor") -> ("Value"=w436:dbl)  [unwired: 1 out]
        n272 = Select(t=w436, s=w437, f=0.0) -> (s? t:f=w434:dbl)
        n273 = call <vilib>:"NT Write Number.vi"("Numeric"=w434, "Name"=w433) -> ()  [unwired: 9 in, 1 out]
      }
      event "Test Slider": Value Change {
        # "When the test mode slider helper is set, update that\ntree row item's value"
        n274 = event-data() -> ("NewVal"=w441:dbl)  [unwired: 1 in]
        n275 = call <vilib>:"NT Write Number.vi"("Numeric"=w441, "Name"=w442) -> ()  [unwired: 9 in, 1 out]
      }
      event "On/Off": Value Change {
        # "When the test mode on/off helper value is set, update that\ntree row item's value"
        n276 = event-data() -> ("NewVal"=w447:bool)  [unwired: 1 in]
        n277 = Boolean To (0,1)(Boolean=w447) -> (0, 1=w446:i16)
        n278 = call <vilib>:"NT Write Number.vi"("Numeric"=w446, "Name"=w445) -> ()  [unwired: 9 in, 1 out]
      }
      event "Rev/Fwd": Value Change {
        # "When the test mode helper value for relays is set, update that\ntree row item's value"
        n279 = event-data() -> ("NewVal.Forward"=w456:bool, "NewVal.Reverse"=w455:bool)  [unwired: 1 in]
        n280 = Boolean To (0,1)(Boolean=w456) -> (0, 1=w452:i16)
        n281 = Boolean To (0,1)(Boolean=w455) -> (0, 1=w454:i16)
        n282 = Negate(x=w454) -> (-x=w453:i16)
        n283 = Add(x=w452, y=w453) -> (x+y=w451:i16)
        n284 = call <vilib>:"NT Write Number.vi"("Numeric"=w451, "Name"=w450) -> ()  [unwired: 9 in, 1 out]
      }
      event "Test Ring": Value Change {
        # "When a test mode helper value is selected from the ring,\nset the tree item's variable to the string value"
        n285 = event-data() -> ("NewVal"=w461:u16)  [unwired: 1 in]
        n286 = property on="Test Ring" class="Ring (strict)"() -> ("Strings []"=w462:string[])  [unwired: 2 in, 2 out]
        n287 = Index Array(array=w462, index=w461) -> (element=w460:string)
        n288 = call <vilib>:"NT Write String.vi"("String"=w460, "Name"=w459) -> ()  [unwired: 9 in, 1 out]
      }
      event "Rec Mode": Value Change {
        # "Update globals for recording mode and path to read log from.\nClear when logging and let NetworkTables set path for vision to\nuse."
        n289 = event-data() -> ("NewVal"=w474:enum32{"Stop", "Record", "Playback"})  [unwired: 1 in]
        n290 = global write "WPI_DashboardLogging Global.vi" "Logging Filename"(path "") -> ()
        n291 = global write "WPI_DashboardLogging Global.vi" "Recording"(w474) -> ()
        n292 = case shown="\"Playback\"" w474 {
          tunnel: w473 -> [_ w476 w485]
          tunnel: [_ _ w484] -> w470
          tunnel: [_ _ w483] -> _
          tunnel: w468 -> [_ _ w481]
          tunnel: cluster{i32, i32} {-250, 170} -> [_ _ w480]
          tunnel: [_ _ T23 {"Image Size"=TRUE, "Image Type"=TRUE, "Pixel Value"=TRUE, "ROI Information"=TRUE, "Zoom Factor"=FALSE} ("Image Information Shown:All Elements")] -> w466
          tunnel: [_ _ TRUE ("Zoom Factor")] -> w465
          tunnel: w464 -> [_ _ w477]
          frame Default {
          }
          frame "Stop", "Record" {
            # "Place Window too"
            n293 = invoke class="VI" method="FP.Close"(reference=w476) -> (reference out=w475:refnum<vi>)  [unwired: 2 in, 2 out]
            n294 = invoke class="VI" method="Abort VI"(reference=w475) -> ()  [unwired: 2 in, 3 out]
          }
          frame "Playback" {
            n295 = call "Open Playback Panel.vi"("Offset"=w480, "DB VI Ref"=w481, "Playback in"=w485) -> ("Playback out"=w482:refnum<vi>)  [unwired: 8 in]
            n296 = register-events(w482, w477) -> (reference out=w484:refnum<event-registration>, error out=w483:errorcluster)  [unwired: 2 in]
          }
        }
        n297 = property on="Camera Image" class="ImageControl"("Image Information Shown"=w466, "Image Information Visible"=w465) -> ()  [unwired: 2 in, 2 out]
        n298 = call <vilib>:"WPI_DashboardNT Log FieldName Cache.vi"("Operation"=enum16{"Lookup/Add", "Index", "Clear"}."Clear") -> ()  [unwired: 8 in, 3 out]
      }
      event Panel Close {
        w487 = enum32{"Stop", "Record", "Playback"}."Stop" ("Rec Mode")
        # "Playback window has been closed, abort"
        n299 = event-data() -> ()  [unwired: 1 in, 4 out]
        n300 = local write "Rec Mode"(w487) -> ()
        n301 = global write "WPI_DashboardLogging Global.vi" "Recording"(w487) -> ()
      }
      event Panel Close {
        # "Abort playback window and ourself"
        n302 = event-data() -> ()  [unwired: 1 in, 4 out]
        n303 = invoke class="VI" method="FP.Close"(reference=w493) -> (reference out=w492:refnum<vi>)  [unwired: 2 in, 2 out]
        n304 = invoke class="VI" method="Abort VI"(reference=w492) -> (error out=w491:errorcluster)  [unwired: 2 in, 2 out]
        n305 = invoke class="VI" method="Abort VI"(error in=w491) -> ()  [unwired: 2 in, 3 out]
      }
      event User Event {
        n306 = event-data() -> ("IDs"=w501:cluster{"RPC field ID":u16, "Unique ID":u16}, "String"=w500:string)  [unwired: 1 in]
        n307 = Bundle("IDs"=w501, "String"=w500) -> (w499:T9)  [unwired: 1 in]
        n308 = call <vilib>:"Retrieve RPC Response.vi"("RPC Response"=w499) -> ("Output"=w496:string[][])  [unwired: 10 in]
        n309 = Build Array (concatenate)(w494, w496) -> (w495:string[][])
        n310 = local write "Command Params"(w495) -> ()
        n311 = local write "Cmd Status"("" ("Cmd Status")) -> ()
      }
      event "Vision": Value Change {
        # "Enable/Disable Compression slider.\nHW USB is hard-coded into the camera"
        n312 = event-data() -> ("NewVal"=w508:u16)  [unwired: 1 in]
        n313 = Equal?(x=w508, y=u32 2 ("milliseconds to wait")) -> (x = y?=w506:bool)
        n314 = Select(t=T24."Disabled and Grayed Out" ("Disabled"), s=w506, f=T24."Enabled" ("Disabled")) -> (s? t:f=w503:T24)
        n315 = property on="Compression" class="Slide (strict)"("DisabledEnum"=w503) -> ()  [unwired: 2 in, 2 out]
      }
      event "Tree": Double Click {
        n316 = event-data() -> ("PlatMods"=w513:T27, "Tag"=w512:string)  [unwired: 1 in]
        n317 = Unbundle(w513) -> ("Shift"=w511:bool)  [unwired: 4 out]
        n318 = Not(x=w511) -> (.not. x?=w510:bool)
        n319 = call <vilib>:"NT Update Persistence.vi"("Persistence"=w510, "Name"=w512) -> ()  [unwired: 9 in, 1 out]
      }
    }
  }
  n320 = while {
    tunnel: w47 -> [w517]
    i -> [w520]
    stop <- FALSE stop-if-true
    n321 = Wait (ms)(milliseconds to wait=u32 100) -> ()  [unwired: 1 out]
    n322 = case shown="\"Playback\"" "Rec Mode" {
      tunnel: w520 -> [_ _ w535]
      tunnel: [u32 2829099 ("Base Color") u32 11141120 ("Target Color") w524] -> w516
      frame "Stop", Default {
        # "Reset the color, extra updates don't cost much"
      }
      frame "Record" {
      }
      frame "Playback" {
        # "Playback"
        n323 = Quotient & Remainder(x=w535, y=u32 50 ("milliseconds to wait")) -> (x-y*floor(x/y)=w531:u32)  [unwired: 1 out]
        n324 = Divide(x=w531, y=u32 50 ("milliseconds to wait")) -> (x/y=w528:dbl)
        n325 = Multiply(x=6.283185307179586, y=w528) -> (x*y=w533:dbl)
        n326 = Sine(x=w533) -> (sin(x)=w532:dbl)
        n327 = Absolute Value(x=w532) -> (abs(x)=w525:dbl)
        n328 = call "Interpolate RGB Color.vi"("Proportion"=w525, "Target Color"=u32 30976, "Base Color"=u32 2829099) -> ("Result Color"=w524:u32)  [unwired: 8 in]
      }
    }
    n329 = property class="Pane"(reference=w517, "PaneColor"=w516) -> ()  [unwired: 1 in, 2 out]
  }
  n330 = local write "Dashboard Tab"(T1."Drive" ("Dashboard Tab")) -> ()
  n331 = property on="On/Off" class="Bool (strict)"("Visible"=w15) -> ()  [unwired: 2 in, 2 out]
  n332 = property on="Motor" class="Clust (strict)"("Visible"=w15) -> ()  [unwired: 2 in, 2 out]
  n333 = property on="Progress" class="Clust (strict)"("Visible"=w15) -> ()  [unwired: 2 in, 2 out]
  n334 = property on="Test Ring" class="Ring (strict)"("Visible"=w15) -> ()  [unwired: 2 in, 2 out]
  n335 = property on="Rev/Fwd" class="Clust (strict)"("Visible"=w15) -> ()  [unwired: 2 in, 2 out]
  n336 = property on="Camera Settings" class="Clust (strict)"("Visible"=w15) -> ()  [unwired: 2 in, 2 out]
  n337 = while {
    tunnel: u16 1741 ("timeout ms (25000)") -> [w537]
    stop <- FALSE stop-if-true
    n338 = TCP Create Listener(10:w537) -> (0:w536:errorcluster, 3:w538:refnum<k5>)  [unwired: 4 in, 1 out]
    n339 = case shown="No Error" w536 {
      selector: w536 -> [w540 _]
      tunnel: w538 -> [w541 _]
      frame No Error {
        n340 = while {
          tunnel: w541 -> [w544]
          tunnel: w540 -> [w543]
          stop <- FALSE stop-if-true
          n341 = TCP Wait On Listener(8:w543, 11:w544) -> (0:w545:errorcluster, 4:w546:refnum<k5>)  [unwired: 2 in, 3 out]
          n342 = local write "TCP"(w546) -> ()
          n343 = case shown="No Error" w545 {
            frame No Error {
            }
            frame Error {
              n344 = Wait (ms)(milliseconds to wait=u32 1000) -> ()  [unwired: 1 out]
            }
          }
        }
      }
      frame Error {
        n345 = Wait (ms)(milliseconds to wait=u32 1000) -> ()  [unwired: 1 out]
      }
    }
  }
  n346 = local write "DB Camera Config"(w15) -> ()
  n347 = local write "Command Params"(string[][] [] ("Command Params")) -> ()
  n348 = global write "WPI_DashboardLogging Global.vi" "Recording"(w41) -> ()
  n349 = local write "Command Selection"(u16 0 ("milliseconds to wait")) -> ()
  n350 = local write "Rec Mode"(w41) -> ()
